vi "Get TipText.vi"(8 "error in (no error)":errorcluster, 11 "object in":refnum<class "Vi_Button.lvclass">) -> (0 "error out":errorcluster, 2 "TipText":string, 3 "object out":refnum<class "Vi_Button.lvclass">)   [LabVIEW 2018, in "Vi_Button.lvclass"]
doc: "Override the Get Tip Text method to generate the tip from the vi's description or name if the description is empty."
uses:
  Vi_Button.lvclass
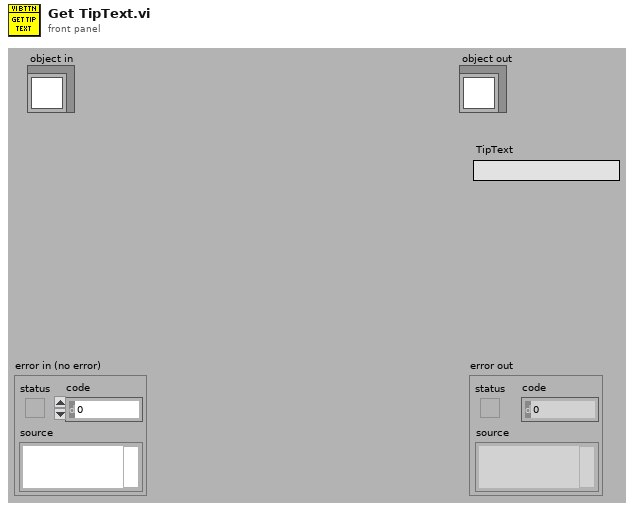
[diagram p1: front panel]
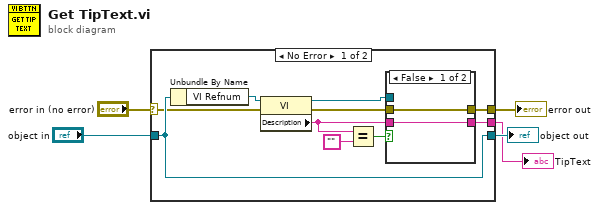
[diagram p0: block diagram]
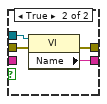
[diagram p2: hidden frame]
diagram:
  n1 = case shown="No Error" "error in (no error)" {
    selector: "error in (no error)" -> [w7 w23]
    tunnel: [w6 w23] -> w4
    tunnel: [w15 w22] -> w2
    tunnel: "object in" -> [w15 w22]
    tunnel: [w9 _] -> w1
    frame No Error {
      n2 = Unbundle By Name(w15) -> ("VI Refnum"=w14:refnum<vi>)
      n3 = property class="VI"(reference=w14, error in=w7) -> (reference out=w11:refnum<vi>, error out=w10:errorcluster, "Description"=w8:string)
      n4 = Equal?(x=w8, y="") -> (x = y?=w12:bool)
      n5 = case shown="False" w12 {
        tunnel: w11 -> [_ w21]
        tunnel: w10 -> [w16 w20]
        tunnel: [w17 w19] -> w9
        tunnel: w8 -> [w17 _]
        tunnel: [w16 w18] -> w6
        frame False {
        }
        frame True {
          n6 = property class="VI"(reference=w21, error in=w20) -> (error out=w18:errorcluster, "Name"=w19:string)  [unwired: 1 out]
        }
      }
    }
    frame Error {
    }
  }
  "error out" <- w4
  "object out" <- w2
  "TipText" <- w1
